vi "read_para_portU32.vi"(11 "address":i16=888 caption="地址" format="%.0x") -> (2 "数据线读取":bool, 3 "IO connector":T1 caption="IO连接器")   [LabVIEW 2011]
uses:
  <vilib>/Platform/portaccess.llb/In Port32.vi
panel:
  # "DB25\tport\tread/write\t反转逻辑\n1   \t16     \tW\t         是\n2\t   0      \tR&W\t       否\n3\t   1\t      R&W\t       否\n4\t\t  2\t\t     R&W\t       否\n5\t\t  3\t\t     R&W\t\t      否\n6\t\t  4\t     \tR&W\t\t      否\n7\t\t  5\t\t     R&W\t\t      否\n8\t   6\t      R&W\t       否\n9\t   7\t      R&W\t       否\n10   14\t     R\t         否\n11\t  15\t     R\t         是\n12  \t13     \tR\t         否\n13\t  12     \tR\t         否\n14\t  17\t     W\t         是\n15\t  11     \tR\t         否\n16\t  18\t     W         \t否\n17\t  19\t     W\t         是\n18\t  20\t    GND\t\n19\t  21\t    GND\t\n20  \t22    \tGND\t\n21  \t23    \tGND\t\n22\t  24\t    GND\t\n23  \t10    \tGND\t\n24  \t9     \tGND\t\n25  \t8     \tGND"
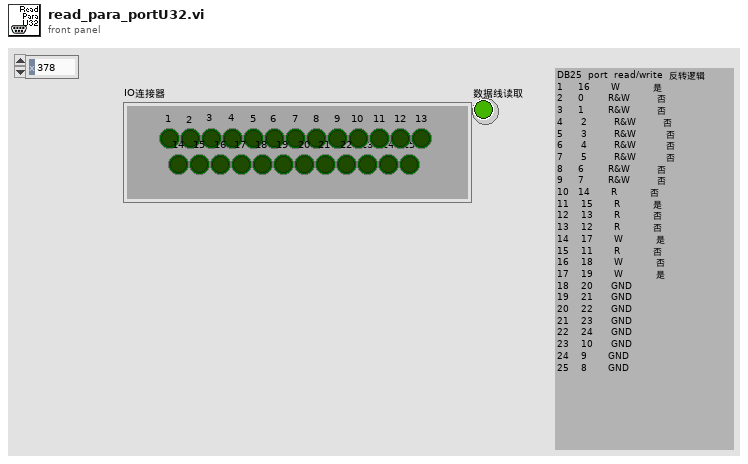
[diagram p1: front panel]
types:
  T1 = cluster{"2":bool, "3":bool, "4":bool, "5":bool, "6":bool, "7":bool, "8":bool, "9":bool, "25":bool, "24":bool, "23":bool, "15":bool, "13":bool, "12":bool, "10":bool, "11":bool, "1":bool, "14":bool, "16":bool, "17":bool, "18":bool, "19":bool, "20":bool, "21":bool, "22":bool}
  T2 = cluster{"D0":bool, "D1":bool, "D2":bool, "D3":bool, "D4":bool, "D5":bool, "D6":bool, "D7":bool, "GND8":bool, "GND7":bool, "GND6":bool, "nError":bool, "Select":bool, "PaperEnd":bool, "nAck":bool, "Busy":bool, "nStrobe":bool, "nAutoLF":bool, "nInit":bool, "nSelectIN":bool, "GND0":bool, "GND1":bool, "GND2":bool, "GND3":bool, "GND4":bool}
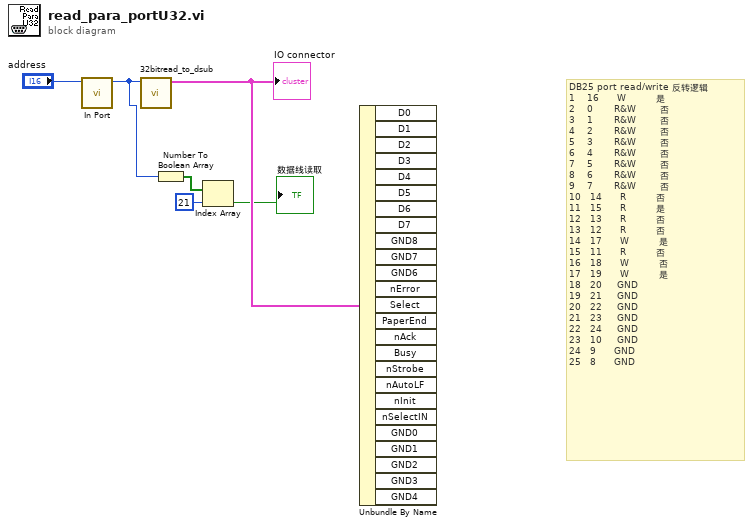
[diagram p0: block diagram]
diagram:
  # "DB25\tport\tread/write\t反转逻辑\n1   \t16     \tW\t         是\n2\t   0      \tR&W\t       否\n3\t   1\t      R&W\t       否\n4\t\t  2\t\t     R&W\t       否\n5\t\t  3\t\t     R&W\t\t      否\n6\t\t  4\t     \tR&W\t\t      否\n7\t\t  5\t\t     R&W\t\t      否\n8\t   6\t      R&W\t       否\n9\t   7\t      R&W\t       否\n10   14\t     R\t         否\n11\t  15\t     R\t         是\n12  \t13     \tR\t         否\n13\t  12     \tR\t         否\n14\t  17\t     W\t         是\n15\t  11     \tR\t         否\n16\t  18\t     W         \t否\n17\t  19\t     W\t         是\n18\t  20\t    GND\t\n19\t  21\t    GND\t\n20  \t22    \tGND\t\n21  \t23    \tGND\t\n22\t  24\t    GND\t\n23  \t10    \tGND\t\n24  \t9     \tGND\t\n25  \t8     \tGND"
  n1 = call-poly <vilib>:"In Port.vi"("address"="address") -> ("data read"=w4:i32)  [unwired: 7 in, 1 out]
  n2 = call "32bitread_to_dsub.vi"("data in"=w4) -> ("IO connector"=w5:T2)  [unwired: 1 in, 7 out]
  "IO connector" <- w5
  n3 = Number To Boolean Array(number=w4) -> (Boolean array=w3:bool[])
  n4 = Index Array(array=w3, index=21 ("索引")) -> (element=→"数据线读取":bool)
  n5 = Unbundle By Name(w5) -> ()  [unwired: 25 out]
